vi "Write Log Line.vi"(10 "log line":string, 11 "handler in":refnum<class "Formatting Handler.lvclass">) -> (0 "error out":errorcluster, 3 "handler out":refnum<class "Formatting Handler.lvclass">)   [LabVIEW 2018, in "Logging.lvlib" / "Formatting Handler.lvclass"]
uses:
  Formatting Handler.lvclass
  <vilib>/ErrorRing/Error Ring.xnode
panel:
  # "Connector Pane"
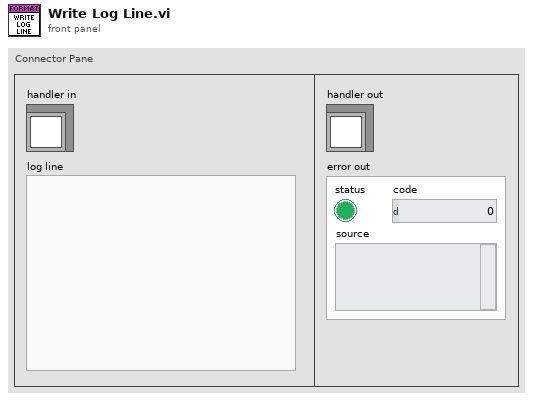
[diagram p1: front panel]
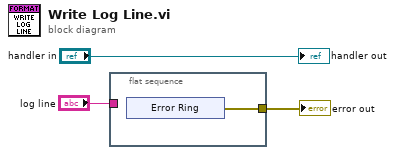
[diagram p0: block diagram]
diagram:
  n1 = flat-sequence {
    tunnel: "log line" -> [_]
    tunnel: [w4] -> w1
    frame #0 {
      n2 = xnode "Error Ring"() -> ("error out"=w4:errorcluster)
    }
  }
  "handler out" <- "handler in"
  "error out" <- w1
